vi "02lee_panel.vi"(1 "Equipo Nº":i32, 2 "Paneles":T1(array[cluster]) {"Nº" min=1.0 max=60.0 step=1.0 format="%#2.1f"; "Ultima recepción" format="%<%d/%m - %X>T"; "Med\nPpal" format="%_4g"}) -> (0 "Panel":T2 {"Ultima recepción" format="%<%d/%m - %X>T"})   [LabVIEW 2010]
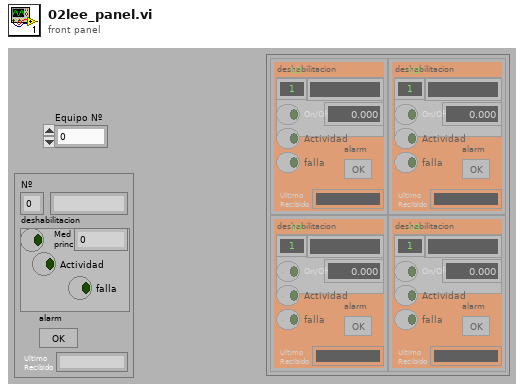
[diagram p1: front panel]
types:
  T1 = cluster{"Nombre":string, "Med\nPpal":dbl, "On/Off":bool, "Ultima recepción":timestamp, "Nº":dbl, "deshabilitacion":bool, "Actividad":bool, "falla":bool, "alarm":bool}[][]
  T2 = cluster{"Nombre":string, "Med\nprinc":dbl, "On/Off":bool, "Ultima recepción":timestamp, "Nº":dbl, "deshabilitacion":bool, "Actividad":bool, "falla":bool, "alarm":bool}
  T3 = cluster{"Nombre":string, "Med\nPpal":dbl, "On/Off":bool, "Ultima recepción":timestamp, "Nº":dbl, "deshabilitacion":bool, "Actividad":bool, "falla":bool, "alarm":bool}
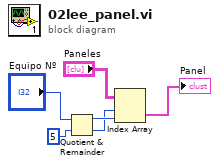
[diagram p0: block diagram]
diagram:
  n1 = Quotient & Remainder(x="Equipo Nº", y=5) -> (x-y*floor(x/y)=w6:i32, floor(x/y)=w5:i32)
  n2 = Index Array(array="Paneles", index (row)=w5, index (col)=w6) -> (element=→"Panel":T3)
